vi "EnumOpenedVIs.vi"(8 "error in (no error)":errorcluster, 11 "Application in":refnum<vi>) -> (0 "error out":errorcluster, 1 "Positions":string[](array[string]), 2 "VI Tags":string[](array[string]), 3 "Application out":refnum<vi>)   [LabVIEW 2019]
uses:
  b5b0ca77-5f3c-4af6-9f2c-4ccc2142e757.vi
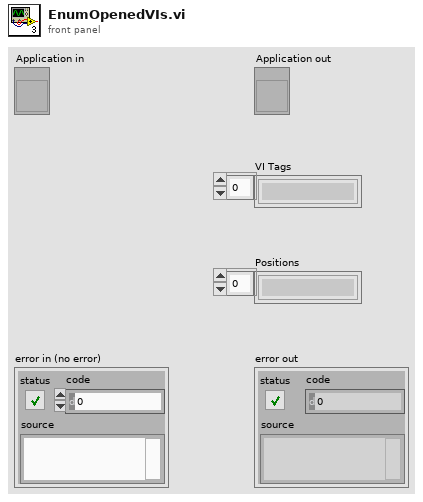
[diagram p1: front panel]
types:
  T1 = enum32{"Bad", "Idle", "Run top level", "Running"}
  T2 = enum32{"Invalid", "Standard", "Closed", "Hidden", "Minimized", "Maximized"}
  T3 = typedef "LVRectTypeDef.ctl" = cluster{"Left":i16, "Top":i16, "Right":i16, "Bottom":i16}
  T4 = enum32{"Bad", "Idle", "Run top level", "Running"}[]
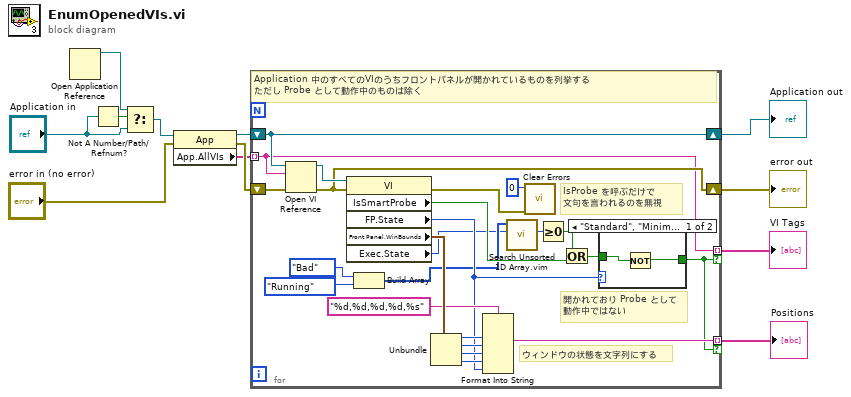
[diagram p0: block diagram]
diagram:
  n1 = Open Application Reference() -> (3:w1:refnum<vi>)  [unwired: 4 in, 1 out]
  n2 = Not A Number/Path/Refnum?(number/path/refnum="Application in") -> (NaN/Path/Refnum?=w4:bool)
  n3 = Select(t=w1, s=w4, f="Application in") -> (s? t:f=w2:refnum<vi>)
  n4 = property class="App"(reference=w2, error in="error in (no error)") -> (reference out=w8:refnum<vi>, error out=w11:errorcluster, "App.AllVIs"=w9:string[])
  n5 = for {
    tunnel: w9 -> [w30] mode=indexing
    shift-right: [w34] -> w12
    shift-left: w11 -> [w35]
    shift-right: [w31] -> w7
    shift-left: w8 -> [w31]
    tunnel: [w30] -> w6 mode=indexing if=w22
    tunnel: [w23] -> w5 mode=indexing if=w22
    # "ウィンドウの状態を文字列にする"
    # "開かれており Probe として\n動作中ではない"
    # "IsProbe を呼ぶだけで\n文句を言われるのを無視"
    # "Application 中のすべてのVIのうちフロントパネルが開かれているものを列挙する\nただし Probe として動作中のものは除く"
    n6 = Open VI Reference(application reference (local)=w31, vi path=w30, error in (no error)=w35) -> (vi reference=w36:refnum<vi>, error out=w34:errorcluster)  [unwired: 3 in]
    n7 = property class="VI"(reference=w36, error in=w34) -> (error out=w33:errorcluster, "IsSmartProbe"=w21:bool, "FP.State"=w20:T2, "Front Panel.WinBounds"=w29:T3, "Exec.State"=w16:T1)  [unwired: 1 out]
    n8 = Build Array(T1."Bad" ("Execution:State"), T1."Running" ("Execution:State")) -> (w17:T4)
    n9 = Unbundle(w29) -> ("Left"=w27:i16, "Top"=w26:i16, "Right"=w25:i16, "Bottom"=w24:i16)
    n10 = Format Into String(format string="%d,%d,%d,%d,%s", w27, w26, w25, w24, w20) -> (resulting string=w23:string)  [unwired: 2 in, 1 out]
    n11 = call "Search Unsorted 1D Array.vim"("element"=w16, "unsorted 1D array"=w17) -> ("index of element"=w15:i32)  [unwired: 9 in]
    n12 = call <vilib>:"Clear Errors.vi"("error in (no error)"=w33, "specific error code to clear (0: all)"=0) -> ()  [unwired: 4 in, 2 out]
    n13 = Greater Or Equal To 0?(x=w15) -> (x >= 0?=w13:bool)
    n14 = Or(x=w13, y=w21) -> (x .or. y?=w14:bool)
    n15 = case shown="\"Standard\", \"Minimized\", \"Maximized\"" w20 {
      tunnel: [w38 _] -> w22
      tunnel: w14 -> [w37 _]
      frame "Standard", "Minimized", "Maximized" {
        n16 = Not(x=w37) -> (.not. x?=w38:bool)
      }
      frame Default {
      }
    }
  }
  "VI Tags" <- w6
  "error out" <- w12
  "Application out" <- w7
  "Positions" <- w5
